vi "SUM.vi"(1 "Max. Number":dbl) -> (0 "Sum":dbl)   [LabVIEW 2015]
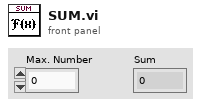
[diagram p1: front panel]
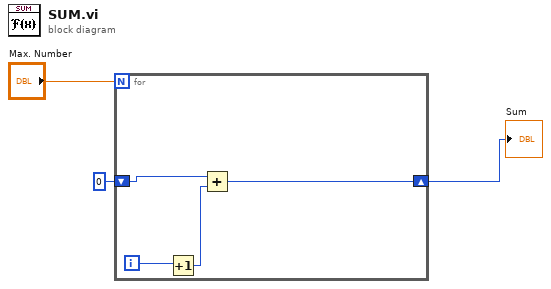
[diagram p0: block diagram]
diagram:
  n1 = for {
    N: "Max. Number" -> [_]
    shift-right: [w5] -> w2
    shift-left: 0 -> [w4]
    i -> [w7]
    n2 = Increment(x=w7) -> (x+1=w6:i32)
    n3 = Add(x=w4, y=w6) -> (x+y=w5:i32)
  }
  "Sum" <- w2
